vi "SIM Detect FuncEval Error.vi"(1 "Simulation data":T1={"continuous integrator"=enum."RK 1 (Euler)", "initial time"=0.0, "final time"=0.0, "step size"=0.0, "proposed step size"=0.0, "max step size"=0.0, "min step size"=0.0, "discrete time step"=0.0, "max step ratio"=0.0, "Diag Eval Stage"=enum."Init", "Substep Index"=0, "Timestep Index"=0.0, "simulation time"=0.0, "current timestep base"=0.0, "proposed step time"=0.0, "absolute tolerance"=0.0, "relative tolerance"=0.0, "step accepted?"=FALSE, "step complete?"=FALSE, "Halt?"=FALSE, "reset integrator?"=FALSE, "machine epsilon"=0.0, "min float"=0.0, "error"={"status"=FALSE, "code"=0, "source"=""}, "Method Order"=0, "Finished Late [i-1]"=FALSE, "Discrete step?"=FALSE, "NaN and Inf check?"=FALSE, "Final Timestep Index"=0.0, "(maj+disc)or(init)?"=FALSE, "Full Solver Reset"=TRUE, "Execution Mode"=enum."Simulate to Completion", "check vector sizes?"=FALSE, "solver handles zc?"=FALSE, "Simulation Registry"={"Current Idx"=0, "Node Tags"=[], "Node Headers"=[], "Node Data"=[], "Cont State data"={"inputs"=[], "outputs"=[], "reset"=[], "lower limits"=[], "upper limits"=[], "limit types"=[], "reset types"=[], "initial conditions"=[], "reset I.C."=[], "limited?"=[], "State Names"=[]}, "DiscreteInfo"={"tick period (sec)"=0.0, "time (ticks)"=0, "fire?"=[], "registry"={"period (sec)"=[], "skew (sec)"=[], "period (tick)"=[], "skew (tick)"=[]}, "discrete \nblocks?"=FALSE, "steps per tick"=0.0, "steps to tick"=0.0, "discrete \ntick?"=FALSE}, "Disc State data"={"Disc States"=[], "State Names"=[]}, "Registry Error"={"Error Block ID"=0, "code"=0}, "ZC Indices"=[]}, "variable step solver?"=FALSE, "First Substep?"=FALSE, "Continuous States?"=FALSE} {"min float" format="%.1e"; "proposed step size" format="%.1e"; "proposed step time" format="%.1e"; "max step ratio" format="%.1e"; "min step size" format="%.1e"; "machine epsilon" format="%.1e"; "discrete time step" format="%.1e"; "max step size" format="%.1e"; "current timestep base" format="%.1e"; "final time" format="%.1e"; "simulation time" format="%.1e"; "relative tolerance" format="%.1e"; "absolute tolerance" format="%.1e"; "Substep Index" format="%.1e"; "step size" format="%.1e"; "initial time" format="%.1e"}) -> (0 "Simulation data out":T1={"continuous integrator"=enum."RK 1 (Euler)", "initial time"=0.0, "final time"=0.0, "step size"=0.0, "proposed step size"=0.0, "max step size"=0.0, "min step size"=0.0, "discrete time step"=0.0, "max step ratio"=0.0, "Diag Eval Stage"=enum."Init", "Substep Index"=0, "Timestep Index"=0.0, "simulation time"=0.0, "current timestep base"=0.0, "proposed step time"=0.0, "absolute tolerance"=0.0, "relative tolerance"=0.0, "step accepted?"=FALSE, "step complete?"=FALSE, "Halt?"=FALSE, "reset integrator?"=FALSE, "machine epsilon"=0.0, "min float"=0.0, "error"={"status"=FALSE, "code"=0, "source"=""}, "Method Order"=0, "Finished Late [i-1]"=FALSE, "Discrete step?"=FALSE, "NaN and Inf check?"=FALSE, "Final Timestep Index"=0.0, "(maj+disc)or(init)?"=FALSE, "Full Solver Reset"=TRUE, "Execution Mode"=enum."Simulate to Completion", "check vector sizes?"=FALSE, "solver handles zc?"=FALSE, "Simulation Registry"={"Current Idx"=0, "Node Tags"=[], "Node Headers"=[], "Node Data"=[], "Cont State data"={"inputs"=[], "outputs"=[], "reset"=[], "lower limits"=[], "upper limits"=[], "limit types"=[], "reset types"=[], "initial conditions"=[], "reset I.C."=[], "limited?"=[], "State Names"=[]}, "DiscreteInfo"={"tick period (sec)"=0.0, "time (ticks)"=0, "fire?"=[], "registry"={"period (sec)"=[], "skew (sec)"=[], "period (tick)"=[], "skew (tick)"=[]}, "discrete \nblocks?"=FALSE, "steps per tick"=0.0, "steps to tick"=0.0, "discrete \ntick?"=FALSE}, "Disc State data"={"Disc States"=[], "State Names"=[]}, "Registry Error"={"Error Block ID"=0, "code"=0}, "ZC Indices"=[]}, "variable step solver?"=FALSE, "First Substep?"=FALSE, "Continuous States?"=FALSE} {"min float" format="%.1e"; "proposed step size" format="%.1e"; "proposed step time" format="%.1e"; "max step ratio" format="%.1e"; "min step size" format="%.1e"; "machine epsilon" format="%.1e"; "discrete time step" format="%.1e"; "max step size" format="%.1e"; "current timestep base" format="%.1e"; "final time" format="%.1e"; "simulation time" format="%.1e"; "relative tolerance" format="%.1e"; "absolute tolerance" format="%.1e"; "Substep Index" format="%.1e"; "step size" format="%.1e"; "initial time" format="%.1e"})   [LabVIEW 2020]
uses:
  <vilib>/Simulation/Implementation/Shared/SIM simulation data.ctl
  <vilib>/Simulation/Implementation/Shared/SIM integration method.ctl
  <vilib>/Simulation/Implementation/Shared/SIM diagram eval stage.ctl
  <vilib>/Simulation/Implementation/Shared/SIMSCR Execution Mode.ctl
  <vilib>/Simulation/Implementation/Shared/SIM Registry.llb/SIM Simulation Registry.ctl
  <vilib>/Simulation/Implementation/Shared/SIM Registry.llb/SIM Registry Node Header.ctl
  <vilib>/Simulation/Implementation/Shared/SIM Registry.llb/SIM Registry Node Record.ctl
  <vilib>/Simulation/Implementation/Shared/SIM trigger type.ctl
  <vilib>/Simulation/Implementation/Shared/SIM solver state data.ctl
  <vilib>/Simulation/Implementation/Shared/SIM limit type.ctl
  <vilib>/Simulation/Implementation/Shared/SIM discrete data.ctl
  <vilib>/Simulation/Implementation/Shared/SIM Discrete state data.ctl
  <vilib>/Simulation/Implementation/Shared/SIM Registry.llb/SIM Simulation Registry Error.ctl
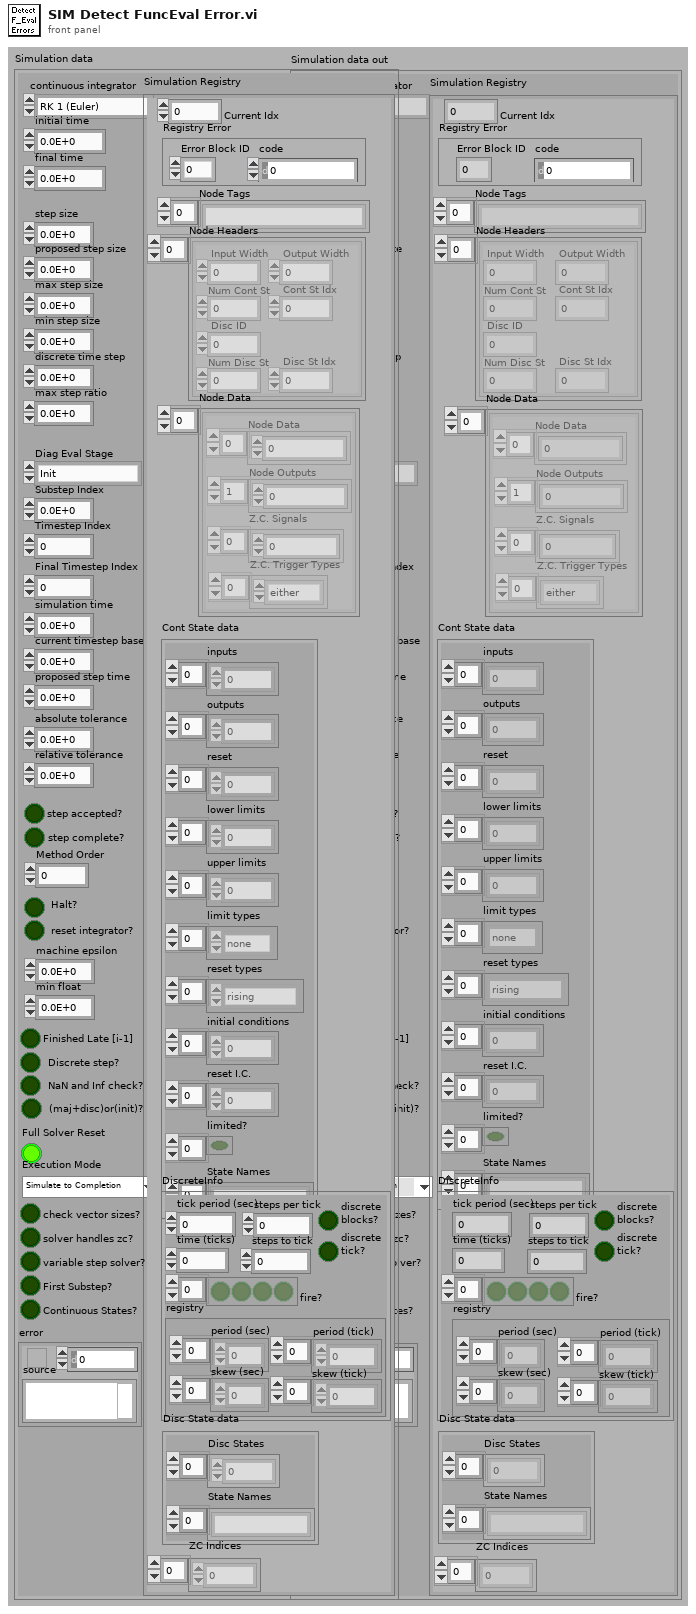
[diagram p1: front panel]
types:
  T1 = typedef "SIM simulation data.ctl" = cluster{"continuous integrator":T2, "initial time":dbl, "final time":dbl, "step size":dbl, "proposed step size":dbl, "max step size":dbl, "min step size":dbl, "discrete time step":dbl, "max step ratio":dbl, "Diag Eval Stage":T3, "Substep Index":i32, "Timestep Index":dbl, "simulation time":dbl, "current timestep base":dbl, "proposed step time":dbl, "absolute tolerance":dbl, "relative tolerance":dbl, "step accepted?":bool, "step complete?":bool, "Halt?":bool, "reset integrator?":bool, "machine epsilon":dbl, "min float":dbl, "error":errorcluster, "Method Order":u32, "Finished Late [i-1]":bool, "Discrete step?":bool, "NaN and Inf check?":bool, "Final Timestep Index":dbl, "(maj+disc)or(init)?":bool, "Full Solver Reset":bool, "Execution Mode":T4, "check vector sizes?":bool, "solver handles zc?":bool, "Simulation Registry":T5, "variable step solver?":bool, "First Substep?":bool, "Continuous States?":bool}
  T2 = typedef "SIM integration method.ctl" = enum16{"RK 1 (Euler)", "Linearizer", "State Query", "Trim Eval", "Adams", "RK 3", "RK 4", "RK 45", "BDF", "RK 2", "RK 23", "Rosenbrock", "Discrete States Only"}
  T3 = typedef "SIM diagram eval stage.ctl" = enum16{"Init", "Minor Substep", "Major Substep", "Final"}
  T4 = typedef "SIMSCR Execution Mode.ctl" = enum16{"Simulate to Completion", "Single Time-Step Simulation (Fixed Step Only)"}
  T5 = typedef "SIM Simulation Registry.ctl" = cluster{"Current Idx":i32, "Node Tags":string[], "Node Headers":T6[], "Node Data":T7[], "Cont State data":T9, "DiscreteInfo":T11, "Disc State data":T12, "Registry Error":T13, "ZC Indices":i32[]}
  T6 = typedef "SIM Registry Node Header.ctl" = cluster{"Input Width":i32, "Disc ID":i32, "Num Cont St":i32, "Cont St Idx":i32, "Num Disc St":i32, "Disc St Idx":i32, "Output Width":i32}
  T7 = typedef "SIM Registry Node Record.ctl" = cluster{"Node Data":dbl[], "Node Outputs":dbl[], "Z.C. Signals":dbl[], "Z.C. Trigger Types":T8[]}
  T8 = typedef "SIM trigger type.ctl" = enum16{"rising", "falling", "either", "none"}
  T9 = typedef "SIM solver state data.ctl" = cluster{"inputs":dbl[], "outputs":dbl[], "reset":dbl[], "lower limits":dbl[], "upper limits":dbl[], "limit types":T10[], "reset types":T8[], "initial conditions":dbl[], "reset I.C.":dbl[], "limited?":bool[], "State Names":string[]}
  T10 = typedef "SIM limit type.ctl" = enum16{"upper", "lower", "both", "none"}
  T11 = typedef "SIM discrete data.ctl" = cluster{"tick period (sec)":dbl, "time (ticks)":i32, "fire?":bool[], "registry":cluster{"period (sec)":dbl[], "skew (sec)":dbl[], "period (tick)":i32[], "skew (tick)":i32[]}, "discrete \nblocks?":bool, "steps per tick":dbl, "steps to tick":dbl, "discrete \ntick?":bool}
  T12 = typedef "SIM Discrete state data.ctl" = cluster{"Disc States":dbl[], "State Names":string[]}
  T13 = typedef "SIM Simulation Registry Error.ctl" = cluster{"Error Block ID":i32, "code":i32}
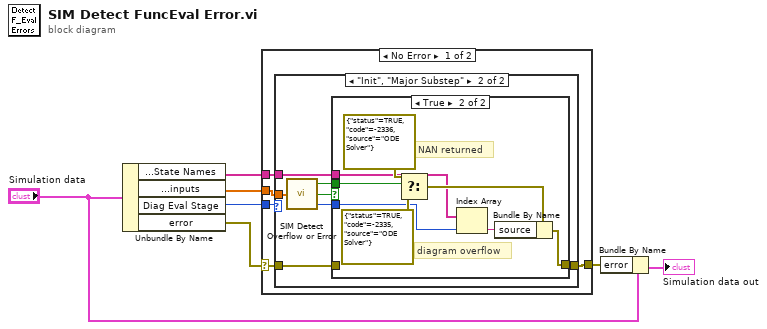
[diagram p0: block diagram]
diagram:
  n1 = Unbundle By Name("Simulation data") -> ("Simulation Registry.Cont State data.State Names"=w6:string[], "Simulation Registry.Cont State data.inputs"=w5:dbl[], "Diag Eval Stage"=w2:T3, "error"=w1:errorcluster)
  n2 = case shown="No Error" w1 {
    selector: w1 -> [w8 w30]
    tunnel: w6 -> [w12 _]
    tunnel: w5 -> [w11 _]
    tunnel: [w10 w30] -> w3
    tunnel: w2 -> [w9 _]
    frame No Error {
      n3 = case shown="\"Init\", \"Major Substep\"" w9 {
        tunnel: [w13 w17] -> w10
        tunnel: w12 -> [_ w16]
        tunnel: w11 -> [_ w15]
        tunnel: w8 -> [w13 w14]
        frame Default {
        }
        frame "Init", "Major Substep" {
          n4 = call <vilib>:"SIM Detect Overflow or Error.vi"("values"=w15) -> ("NaN found?"=w19:bool, "Inf or NaN found?"=w20:bool, "index of Inf or NaN"=w18:i32)
          n5 = case shown="True" w20 {
            tunnel: w19 -> [_ w25]
            tunnel: w18 -> [_ w27]
            tunnel: [w21 w23] -> w17
            tunnel: w16 -> [_ w22]
            tunnel: w14 -> [w21 _]
            frame False {
            }
            frame True {
              # "diagram overflow"
              # "NAN returned"
              n6 = Select(t=errorcluster {"status"=TRUE, "code"=-2336, "source"="ODE Solver"} ("error"), s=w25, f=errorcluster {"status"=TRUE, "code"=-2335, "source"="ODE Solver"} ("error")) -> (s? t:f=w26:errorcluster)
              n7 = Index Array(array=w22, index=w27) -> (element=w24:string)
              n8 = Bundle By Name(cluster=w26, "source"=w24) -> (w23:errorcluster)
            }
          }
        }
      }
    }
    frame Error {
    }
  }
  n9 = Bundle By Name(cluster="Simulation data", "error"=w3) -> (→"Simulation data out":T1)
